vi "addResultsToQ.vi"(8 "error in (no error)":errorcluster, 10 "Results":variant, 11 "ImageAnalyser in":refnum<class "ImageAnalyser.lvclass">) -> (0 "error out":errorcluster, 3 "ImageAnalyser out":refnum<class "ImageAnalyser.lvclass">)   [LabVIEW 2011, in "Tools.lvlib" / "Imaging.lvlib" / "ImageAnalyser.lvclass"]
uses:
  ImageAnalyser.lvclass
panel:
  # "I disabled this!"
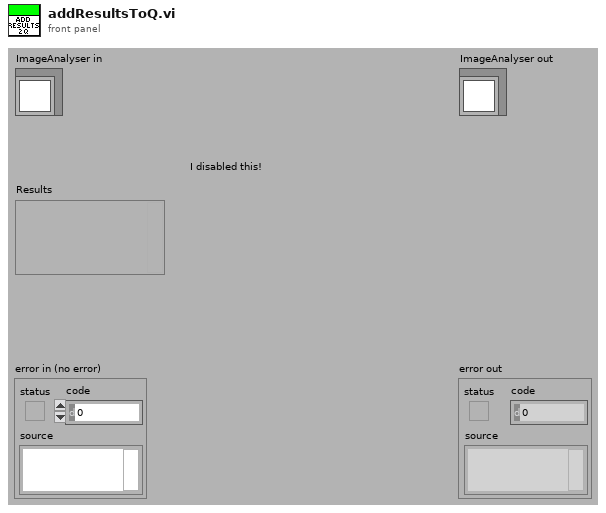
[diagram p1: front panel]
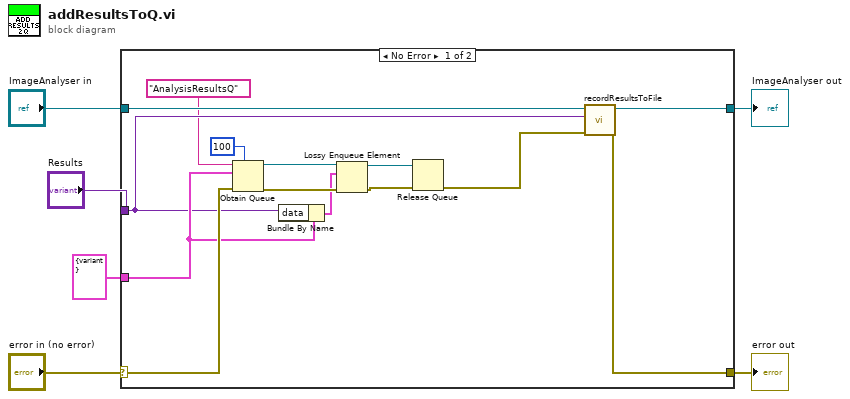
[diagram p0: block diagram]
diagram:
  n1 = case shown="No Error" "error in (no error)" {
    selector: "error in (no error)" -> [w20 w22]
    tunnel: [w15 w22] -> w5
    tunnel: [w17 w21] -> w3
    tunnel: "ImageAnalyser in" -> [w18 w21]
    tunnel: "Results" -> [w16 _]
    tunnel: cluster{"data":variant} {"data"=variant} ("dataQ") -> [w19 _]
    frame No Error {
      n2 = Obtain Queue(max queue size (-1, unlimited)=100, name (unnamed)="AnalysisResultsQ", element data type=w19, error in (no error)=w20) -> (queue out=w13:refnum<queue>, error out=w12:errorcluster)  [unwired: 1 in, 1 out]
      n3 = Bundle By Name(cluster=w19, "data"=w16) -> (w9:cluster{"data":variant})
      n4 = Lossy Enqueue Element(queue=w13, element=w9, error in (no error)=w12) -> (queue out=w11:refnum<queue>, error out=w10:errorcluster)  [unwired: 2 out]
      n5 = Release Queue(queue=w11, error in (no error)=w10) -> (error out=w8:errorcluster)  [unwired: 1 in, 2 out]
      n6 = call-dynamic "recordResultsToFile.vi"("error in (no error)"=w8, "Results"=w16, "ImageAnalyser in"=w18) -> ("error out"=w15:errorcluster, "ImageAnalyser out"=w17:refnum<class "ImageAnalyser.lvclass">)  [unwired: 7 in]
    }
    frame Error {
    }
  }
  "error out" <- w5
  "ImageAnalyser out" <- w3
